vi "TEST.vi"() -> ()   [LabVIEW 2019]
uses:
  D:/SOFT_REPO_GUM/renishawxl80sdk/Dllx64/ComDX10Adaptor.dll
  SOFT_REPO_GUM/renishawxl80sdk/Dllx64/ComDX10Adaptor.dll
panel:
  out "status":i32(ring) items=["Ok"=0, "BadReading"=1, "Failed"=2, "NotConnected"=4]
  out "GetAirTemp":dbl
  out "ConnectLaser":bool
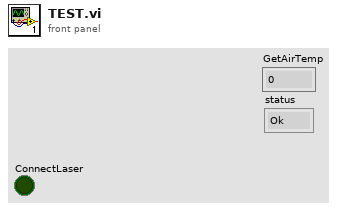
[diagram p1: front panel]
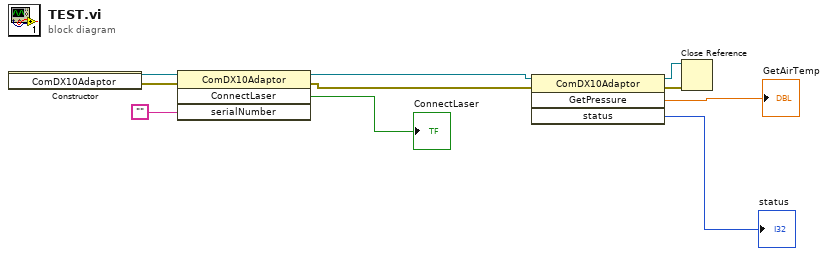
[diagram p0: block diagram]
diagram:
  n1 = constructor class="ComDX10Adaptor"() -> (reference out=w10:refnum<k24>, error out=w9:errorcluster)  [unwired: 3 in, 1 out]
  n2 = invoke class="ComDX10Adaptor" method="ConnectLaser"(reference=w10, error in=w9, "serialNumber"="") -> (reference out=w6:refnum<k24>, error out=w5:errorcluster, "ConnectLaser"=→"ConnectLaser":bool)  [unwired: 1 in, 1 out]
  n3 = invoke class="ComDX10Adaptor" method="GetPressure"(reference=w6, error in=w5) -> (reference out=w1:refnum<k24>, error out=w2:errorcluster, "GetPressure"=→"GetAirTemp":dbl, "status"=→"status":i32)  [unwired: 2 in]
  n4 = Close Reference(reference=w1, error in (no error)=w2) -> ()  [unwired: 1 out]
